vi "Date_Time to String.vi"() -> (3 "date/time string":string)   [LabVIEW 2015, in "Generic Module Library.lvlib" / "Template G_Module.lvlib"]
uses:
  Template G_Module.lvlib
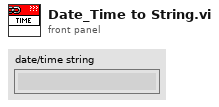
[diagram p1: front panel]
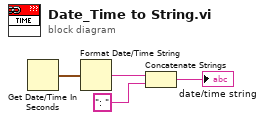
[diagram p0: block diagram]
diagram:
  n1 = Get Date/Time In Seconds() -> (seconds since 1Jan1904=w4:timestamp)
  n2 = Format Date/Time String(seconds (now)=w4) -> (date/time string=w3:string)  [unwired: 2 in]
  n3 = Concatenate Strings(w3, ": " ("string")) -> (→"date/time string":string)
